vi "PlugInInit.vi"(8 "error in (no error)":errorcluster, 11 "Enum":enum16{"Осциллограммы", "ВАХ"}(ring)) -> (0 "error out":errorcluster, 3 "PlugIn_VI_out":refnum<vi>)   [LabVIEW 2012]
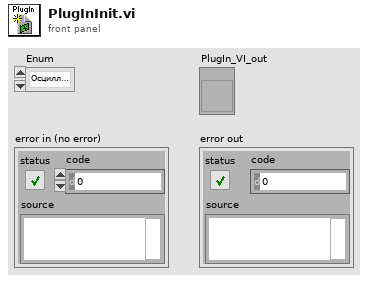
[diagram p1: front panel]
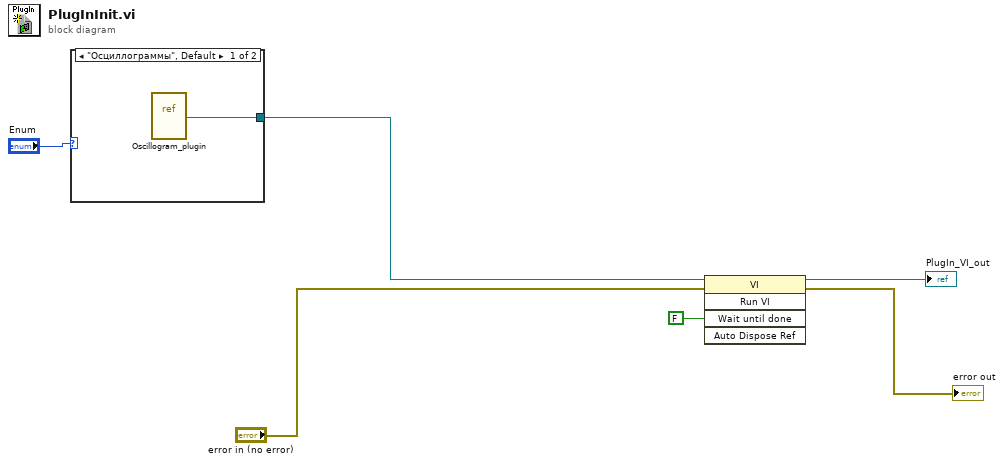
[diagram p0: block diagram]
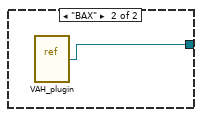
[diagram p2: hidden frame]
diagram:
  n1 = case shown="\"Осциллограммы\", Default" "Enum" {
    tunnel: [w7 w8] -> w4
    frame "Осциллограммы", Default {
      n2 = vi-ref "Oscillogram_plugin.vi"() -> (w7:refnum<vi>)
    }
    frame "ВАХ" {
      n3 = vi-ref "VAH_plugin.vi"() -> (w8:refnum<vi>)
    }
  }
  n4 = invoke class="VI" method="Run VI"(reference=w4, error in="error in (no error)", "Wait until done"=FALSE) -> (reference out=→"PlugIn_VI_out":refnum<vi>, error out=→"error out":errorcluster)  [unwired: 2 in, 3 out]
